vi "步进电机命令输入与输出.vi"(2 "输入字符串":string, 3 "串口通信端口":refnum<visa-resource-name>) -> (0 "返回字符串":string, 1 "串口通信端口 2":refnum<visa-resource-name>)   [LabVIEW 2018]
panel:
  # "步进电机命令输入与输出"
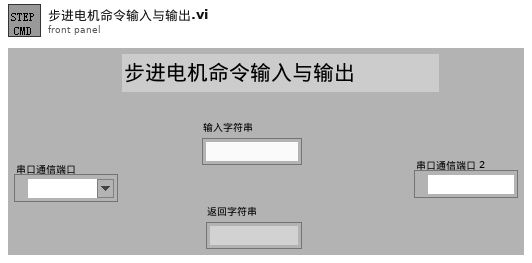
[diagram p1: front panel]
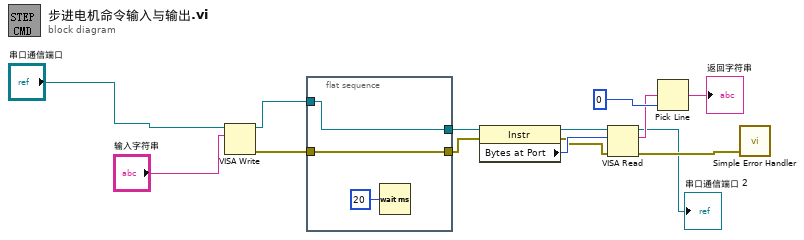
[diagram p0: block diagram]
diagram:
  n1 = VISA Write(VISA resource name="串口通信端口", write buffer="输入字符串") -> (VISA resource name out=w10:refnum<visa-resource-name>, error out=w9:errorcluster)  [unwired: 1 in, 1 out]
  n2 = flat-sequence {
    tunnel: w10 -> [w17]
    tunnel: w9 -> [w16]
    tunnel: [w17] -> w8
    tunnel: [w16] -> w7
    frame #0 {
      n3 = Wait (ms)(milliseconds to wait=u32 20 ("等待时间（毫秒）")) -> ()  [unwired: 1 out]
    }
  }
  n4 = property class="Instr"(reference=w8, error in=w7) -> (reference out=w12:refnum<visa-resource-name>, error out=w11:errorcluster, "Bytes at Port"=w13:u32)
  n5 = VISA Read(VISA resource name=w12, byte count=w13, error in (no error)=w11) -> (VISA resource name out=→"串口通信端口 2":refnum<visa-resource-name>, read buffer=w5:string, error out=w3:errorcluster)  [unwired: 1 out]
  n6 = Pick Line(multi-line string=w5, line index=0 ("行索引")) -> (output string=→"返回字符串":string)  [unwired: 1 out]
  n7 = call <vilib>:"Simple Error Handler.vi"("error in (no error)"=w3) -> ()  [unwired: 1 in, 8 out]
